vi "ExSpectralCalMovCollect.vi"() -> ()   [LabVIEW 2010]
panel:
  out "XY Graph":T1(graph)
  in  "Pixel Width (microns)":dbl format="%.2f"
  in  "Magnification":dbl format="%.2f"
  in  "Detector Angle (degrees)":dbl format="%.2f"
  in  "Inclusion Angle (degrees)":dbl format="%.2f"
  in  "Focal Length (mm)":dbl format="%.2f"
  in  "Slope Adjust":dbl format="%.2f"
  in  "Center Offset":dbl format="%.2f"
  out "Current Wavelength":string
  in  "Increment Wavelength":dbl=50.0 format="%.2f"
  in  "End Wavelength":dbl=700.0 format="%.2f"
  in  "Start Wavelength":dbl format="%.2f"
  in  "Grating Speed":dbl=2000.0 min=1.0 step=1.0 format="%.2f"
  in  "Grating number":i16=1 min=1 max=100 step=1
  in  "Temperature":dbl=-10.0 format="%.2f"
  in  "Exposure":dbl min=0.0 step=0.001 format="%.3f"
  in  "stop":bool
  out "error out":errorcluster
  in  "error in (no error)":errorcluster
  # "ExSpectralCalMovCollect.vi\nCamera and Spectrometer control.  This vi will open both the camera and spectrograph.  It will then move the grating to the Start Wavelength.  Data will then be collected and displayed.  The sequence will be repeated after moving the grating by the Increment Wavelength until the End Wavelength is reached.  At that time, data collection will continue until the STOP button is hit. The display will\nshow an updated calibration in nm."
  # "Calibration Parameters"
  # "NOTES:\nThe properly configured spectrometer .ini file must be present in the LabVIEW folder for spectrograph operation.\n\nConsult the documentation for more information on how to configure these files."
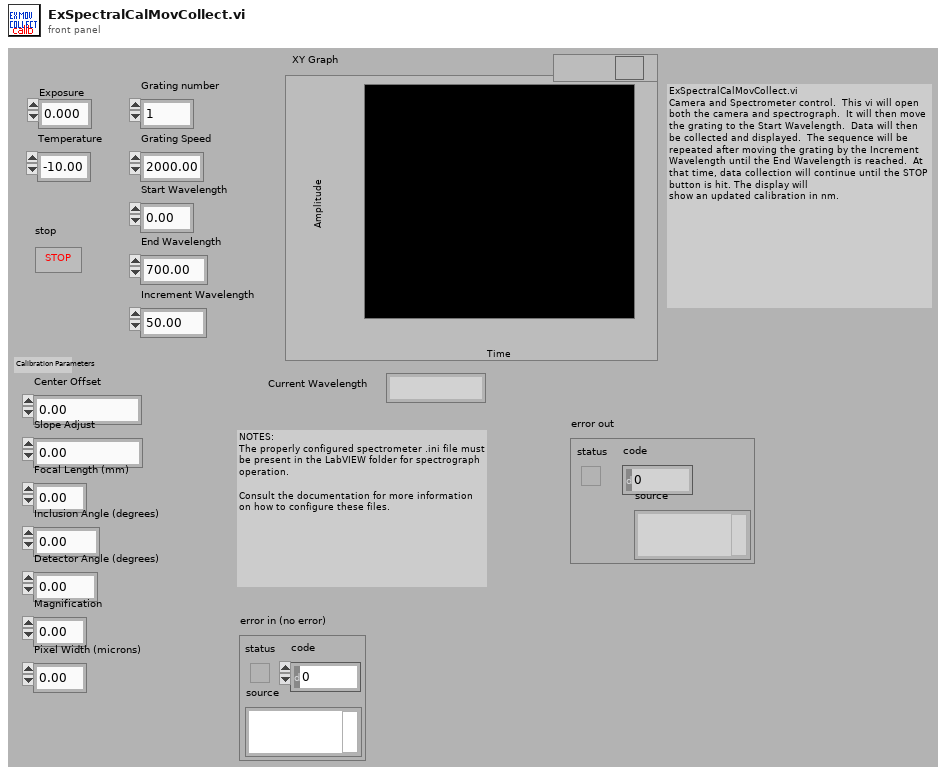
[diagram p1: front panel]
types:
  T1 = cluster{"Calibrated Array":dbl[], "Array F32":sgl[]}
  T2 = cluster{"Center Offset":dbl, "Slope Adjust":dbl, "Focal Length (mm)":dbl, "Inclusion Angle (degrees)":dbl, "Detector Angle (degrees)":dbl, "Magnification":dbl, "Pixel Width (microns)":dbl}
  T3 = cluster{"Camera Handle":u32, "Pulser Handle":u32, "File Handle":u32, "Display Handle":u32, "Image Handle":u32}
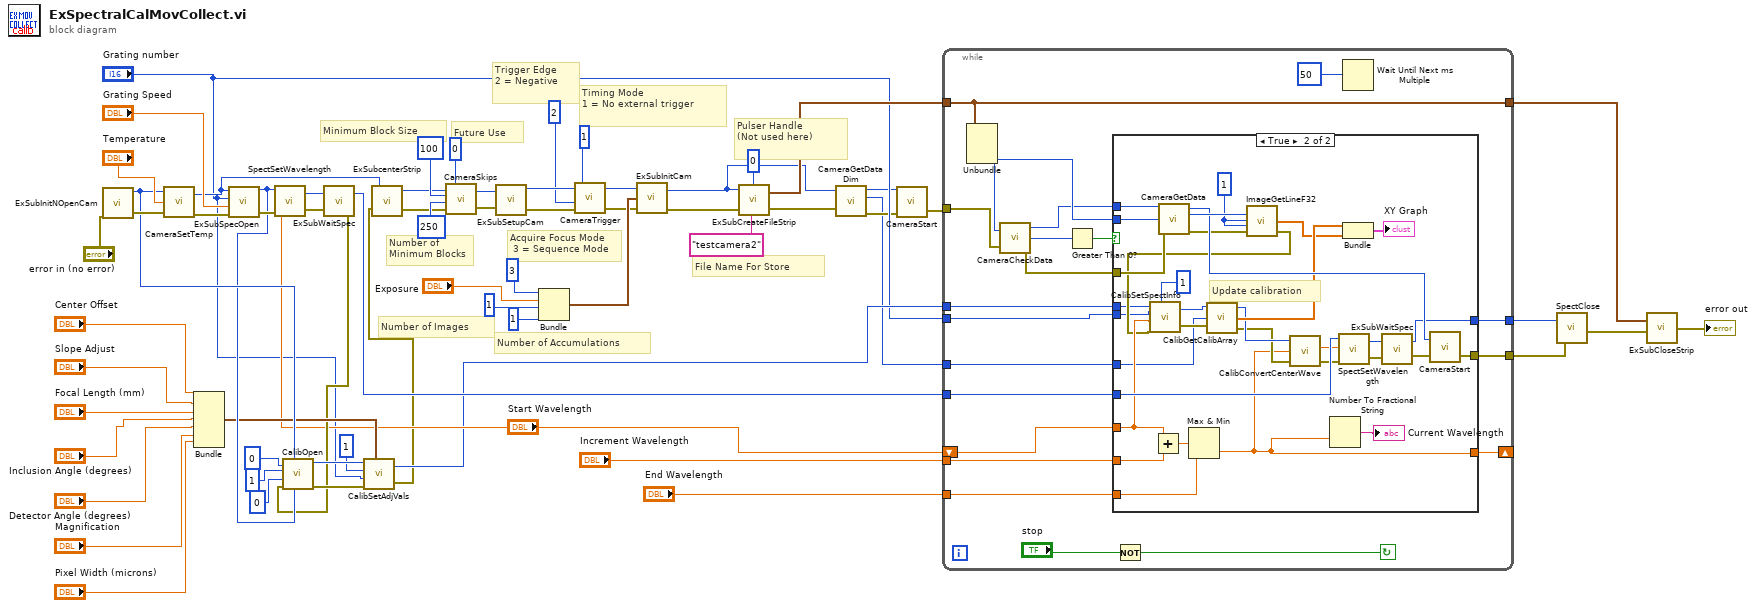
[diagram p0: block diagram]
diagram:
  # "Pulser Handle\n(Not used here)"
  # "Trigger Edge\n2 = Negative"
  # "Timing Mode\n1 = No external trigger"
  # "Future Use"
  # "Number of Minimum Blocks"
  # "Minimum Block Size"
  # "Number of Images"
  # "Number of Accumulations"
  # "Acquire Focus Mode\n 3 = Sequence Mode"
  # "File Name For Store"
  n1 = call "ExSubInitNOpenCam.vi"("error in (no error)"="error in (no error)") -> ("Camera Handle"=w25:u32, "error out"=w29:errorcluster)
  n2 = call <userlib>:"CameraSetTemp.vi"("error in (no error)"=w29, "Temperature"="Temperature", "Camera Handle"=w25) -> ("error out"=w30:errorcluster, "Camera Handle"=w22:u32)
  n3 = Bundle("Center Offset"="Center Offset", "Slope Adjust"="Slope Adjust", "Focal Length (mm)"="Focal Length (mm)", "Inclusion Angle (degrees)"="Inclusion Angle (degrees)", "Detector Angle (degrees)"="Detector Angle (degrees)", "Magnification"="Magnification", "Pixel Width (microns)"="Pixel Width (microns)") -> (w14:T2)  [unwired: 1 in]
  n4 = call "ExSubSpecOpen.vi"("error in (no error)"=w30, "Grating speed"="Grating Speed", "Grating number"="Grating number", "Camera Handles"=w22) -> ("error out"=w35:errorcluster, "Spectrometer Handle"=w23:u32)  [unwired: 1 out]
  n5 = call <userlib>:"SpectSetWavelength.vi"("error in"=w35, "Wavelength"="Start Wavelength", "Spectrometer Handle"=w23) -> ("error out"=w39:errorcluster, "Spectrumeter Handle"=w38:u32)
  n6 = call "ExSubWaitSpec.vi"("error in (no error)"=w39, "Spectrometer Handle"=w38) -> ("error out"=w10:errorcluster, "Spectrometer handle"=w37:u32)
  n7 = call <userlib>:"CalibOpen.vi"("Spectrometer Handle"=w23, "Detector Handle"=w25, "error in"=w10, "Detector Position"=0, "Calibration Type"=1, "Calibration Device ID"=0) -> ("error out"=w12:errorcluster, "Calibration Handle"=w13:u32)
  n8 = call <userlib>:"CalibSetAdjVals.vi"("Calibration Handle"=w13, "Turret Number"=1, "Grating Number"="Grating number", "error in"=w12, "Spectrometer Calibration Parameters"=w14) -> ("Calibration Handle"=w8:u32, "error out"=w6:errorcluster)
  n9 = call "ExSubcenterStrip.vi"("error in (no error)"=w6, "Camera Handle"=w22) -> ("error out"=w41:errorcluster, "Camera Handle"=w42:u32)
  n10 = call <userlib>:"CameraSkips.vi"("Camera Handle"=w42, "Minimum Block Size"=100, "Number of Minimum blocks"=250, "error in"=w41, "Type of Skips"=0) -> ("Camera Handle"=w44:u32, "error out"=w43:errorcluster)
  n11 = call "ExSubSetupCam.vi"("error in (no error)"=w43, "Camera Handle"=w44) -> ("error out"=w49:errorcluster, "Camera Handle"=w53:u32)
  n12 = Bundle(3, "Exposure"="Exposure", 1, 1) -> (w60:cluster{i32, "Exposure":dbl, i32, i32})  [unwired: 1 in]
  n13 = call <userlib>:"CameraTrigger.vi"("error in"=w49, "Trigger Edge"=2, "Timing Mode"=1, "Camera Handle"=w53) -> ("error out"=w54:errorcluster, "Camera Handle"=w52:u32)
  n14 = call "ExSubInitCam.vi"("error in (no error)"=w54, "Camera Information"=w60, "Camera Handle"=w52) -> ("error out"=w59:errorcluster, "Camera Handle"=w5:u32)
  n15 = call "ExSubCreateFileStrip.vi"("error in (no error)"=w59, "File and Display Name"="testcamera2", "Pulser Handle"=0, "Camera Handle"=w5) -> ("error out"=w4:errorcluster, "Handles Out"=w57:T3)
  n16 = call <userlib>:"CameraGetDataDim.vi"("Camera Handle"=w5, "error in"=w4) -> ("Camera Handle"=w2:u32, "Xdim"=w1:u32, "error out"=w3:errorcluster)  [unwired: 1 out]
  n17 = call <userlib>:"CameraStart.vi"("error in"=w3, "Camera Handle"=w2) -> ("error out"=w45:errorcluster)  [unwired: 1 out]
  n18 = while {
    tunnel: w57 -> [w84]
    tunnel: w45 -> [w83]
    tunnel: [w81] -> w31
    tunnel: [w84] -> w56
    tunnel: w37 -> [w75]
    tunnel: "Increment Wavelength" -> [w74]
    tunnel: "End Wavelength" -> [w73]
    shift-right: [w71] -> _
    shift-left: "Start Wavelength" -> [w72]
    tunnel: [w70] -> w32
    tunnel: w8 -> [w69]
    tunnel: "Grating number" -> [w68]
    tunnel: w1 -> [w67]
    stop <- w85 continue-if-true
    n19 = Unbundle(w84) -> ("Camera Handle"=w79:u32, "Image Handle"=w80:u32)  [unwired: 3 out]
    n20 = call <userlib>:"CameraCheckData.vi"("Camera Handle"=w79, "error in"=w83) -> ("Camera Handle"=w78:u32, "Number Of Frames Available"=w76:i32, "error out"=w82:errorcluster)
    n21 = Greater Than 0?(x=w76) -> (x > 0?=w77:bool)
    n22 = case shown="True" w77 {
      tunnel: w82 -> [w90 w123]
      tunnel: [w90 w111] -> w81
      tunnel: w80 -> [_ w120]
      tunnel: w78 -> [_ w119]
      tunnel: w75 -> [w88 w115]
      tunnel: w74 -> [_ w109]
      tunnel: w73 -> [_ w114]
      tunnel: w72 -> [w89 w106]
      tunnel: [w89 w92] -> w71
      tunnel: [w88 w108] -> w70
      tunnel: w69 -> [_ w104]
      tunnel: w68 -> [_ w103]
      tunnel: w67 -> [_ w96]
      frame False {
      }
      frame True {
        w121 = 1
        # "Update calibration"
        n23 = Add(x=w106, y=w109) -> (x+y=w113:dbl)
        n24 = call <userlib>:"CameraGetData.vi"("error in"=w123, "Data Handle"=w120, "Camera Handle"=w119) -> ("error out"=w112:errorcluster, "Data Handle"=w122:u32, "Camera Handle"=w118:u32)
        n25 = Max & Min(x=w113, y=w114) -> (min(x,y)=w92:dbl)  [unwired: 1 out]
        n26 = call <userlib>:"ImageGetLineF32.vi"("error in"=w112, "Z Position"=w121, "Y Position"=w121, "Data Handle"=w122) -> ("error out"=w105:errorcluster, "Array F32"=w98:sgl[])  [unwired: 1 out]
        n27 = call <userlib>:"CalibSetSpectInfo.vi"("Calibration Handle"=w104, "Current Grating Number"=w103, "Current Wavelength"=w106, "error in"=w105, "Current Turret Number"=1) -> ("Calibration Handle"=w100:u32, "error out"=w101:errorcluster)
        n28 = call <userlib>:"CalibGetCalibArray.vi"("error in"=w101, "Array Size"=w96, "Calibration Handle"=w100) -> ("error out"=w94:errorcluster, "Calibrated Array"=w99:dbl[], "Calibration Handle"=w95:u32)
        n29 = call <userlib>:"CalibConvertCenterWave.vi"("error in (no error)"=w94, "Target Center Wavelength"=w92, "Calib Handle"=w95) -> ("error out"=w93:errorcluster, "Spectrometer Wavelength"=w91:dbl)  [unwired: 1 out]
        n30 = Number To Fractional String(number=w92) -> (F-format string=→"Current Wavelength":string)  [unwired: 3 in]
        n31 = call <userlib>:"SpectSetWavelength.vi"("error in"=w93, "Wavelength"=w91, "Spectrometer Handle"=w115) -> ("error out"=w117:errorcluster, "Spectrumeter Handle"=w116:u32)
        n32 = Bundle("Calibrated Array"=w99, "Array F32"=w98) -> (→"XY Graph":T1)  [unwired: 1 in]
        n33 = call "ExSubWaitSpec.vi"("error in (no error)"=w117, "Spectrometer Handle"=w116) -> ("error out"=w107:errorcluster, "Spectrometer handle"=w108:u32)
        n34 = call <userlib>:"CameraStart.vi"("error in"=w107, "Camera Handle"=w118) -> ("error out"=w111:errorcluster)  [unwired: 1 out]
      }
    }
    n35 = Not(x="stop") -> (.not. x?=w85:bool)
    n36 = Wait Until Next ms Multiple(millisecond multiple=50) -> ()  [unwired: 1 out]
  }
  n37 = call <userlib>:"SpectClose.vi"("error in"=w31, "Spectrometer Handle"=w32) -> ("error out"=w33:errorcluster)
  n38 = call "ExSubCloseStrip.vi"("error in (no error)"=w33, "Handles In"=w56) -> ("error out"=→"error out":errorcluster)
